vi "2100_SMU_Meas and Calculate Resitance_No Publish Data.vi"(7 "Current  Level":dbl=-0.01, 8 "error in (no error)":errorcluster, 10 "Pins":string[](array[string]), 11 "Semiconductor Module Context":T1) -> (0 "error Out":errorcluster, 1 "Individual_R_Meas":dbl[](array[numeric]), 3 "Semiconductor Module Context Out":T1)   [LabVIEW 2013]
uses:
  <vilib>/NI_TestStand_SemiconductorModule/NI_TestStand_Semiconductor_Module.lvlibp/PinMap/General/SemiconductorModuleContext.ctl
  <vilib>/NI_TestStand_SemiconductorModule/NI_TestStand_Semiconductor_Module.lvlibp/PinMap/DC Power/PinsToNIDCPowerSessions.vi
  <vilib>/NI_TestStand_SemiconductorModule/NI_TestStand_Semiconductor_Module.lvlibp
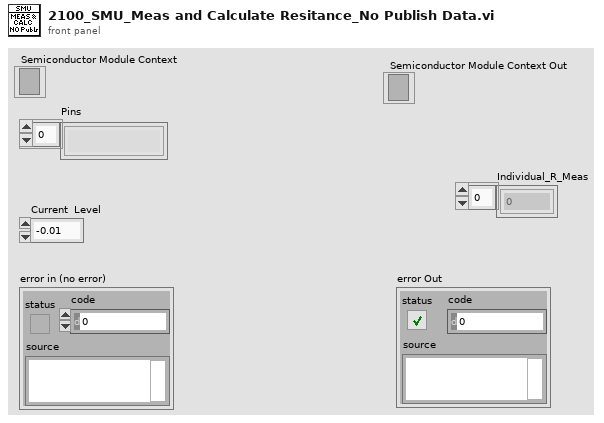
[diagram p1: front panel]
types:
  T1 = typedef "NI_TestStand_Semiconductor_Module.lvlibp/SemiconductorModuleContext.ctl" = refnum<k7>
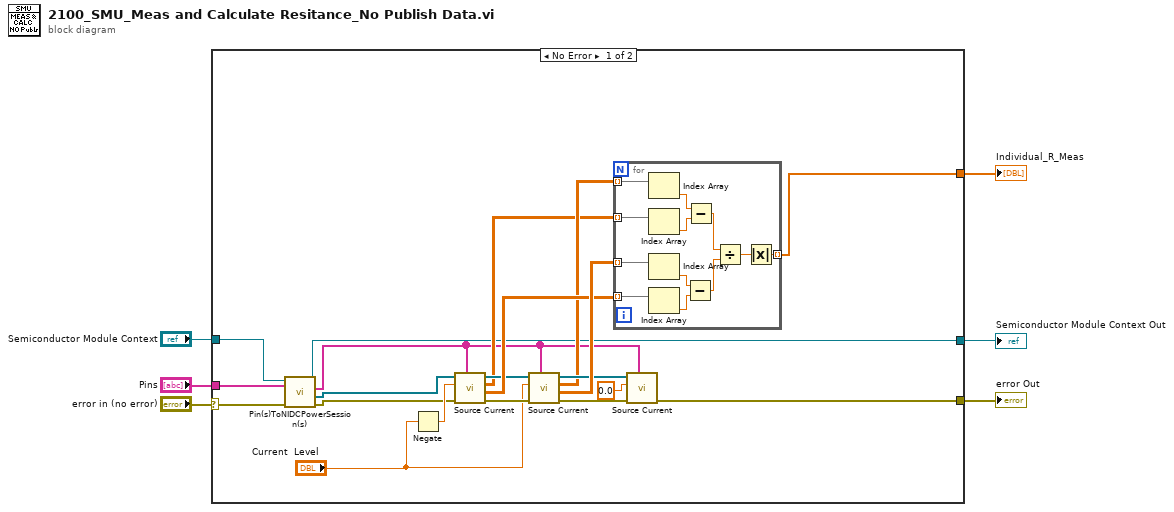
[diagram p0: block diagram]
diagram:
  n1 = case shown="No Error" "error in (no error)" {
    selector: "error in (no error)" -> [w26 w40]
    tunnel: "Semiconductor Module Context" -> [w24 w39]
    tunnel: "Pins" -> [w25 _]
    tunnel: [w10 w40] -> w3
    tunnel: [w9 w39] -> w2
    tunnel: [w7 _] -> w1
    frame No Error {
      n2 = call-poly <vilib>:"Pin(s)ToNIDCPowerSession(s).vi"("error in (no error)"=w26, "Pins"=w25, "Semiconductor Module Context"=w24) -> ("error out"=w12:errorcluster, "Instrument Sessions"=w11:refnum<k15>[], "Channel Lists"=w8:string[], "Semiconductor Module Context Out"=w9:T1)  [unwired: 4 in, 1 out]
      n3 = Negate(x="Current  Level") -> (-x=w20:dbl)
      n4 = call "Source Current.vi"("Channel Lists"=w8, "error in (no error)"=w12, "current level"=w20, "Instrument Sessions In"=w11) -> ("error out"=w18:errorcluster, "current measurements"=w22:dbl[][], "voltage measurements"=w16:dbl[][], "Instrument Sessions Out"=w17:refnum<k15>[])  [unwired: 4 in]
      n5 = call "Source Current.vi"("Channel Lists"=w8, "error in (no error)"=w18, "current level"="Current  Level", "Instrument Sessions In"=w17) -> ("error out"=w15:errorcluster, "current measurements"=w23:dbl[][], "voltage measurements"=w19:dbl[][], "Instrument Sessions Out"=w21:refnum<k15>[])  [unwired: 4 in]
      n6 = for {
        tunnel: w19 -> [w30] mode=indexing
        tunnel: w23 -> [w38] mode=indexing
        tunnel: [w36] -> w7 mode=indexing
        tunnel: w22 -> [w34] mode=indexing
        tunnel: w16 -> [w27] mode=indexing
        n7 = Index Array(array=w30) -> (element=w29:dbl)  [unwired: 1 in]
        n8 = Index Array(array=w27) -> (element=w28:dbl)  [unwired: 1 in]
        n9 = Index Array(array=w38) -> (element=w31:dbl)  [unwired: 1 in]
        n10 = Index Array(array=w34) -> (element=w33:dbl)  [unwired: 1 in]
        n11 = Subtract(x=w31, y=w33) -> (x-y=w32:dbl)
        n12 = Subtract(x=w29, y=w28) -> (x-y=w35:dbl)
        n13 = Divide(x=w35, y=w32) -> (x/y=w37:dbl)
        n14 = Absolute Value(x=w37) -> (abs(x)=w36:dbl)
      }
      n15 = call "Source Current.vi"("Channel Lists"=w8, "error in (no error)"=w15, "current level"=0.0, "Instrument Sessions In"=w21) -> ("error out"=w10:errorcluster)  [unwired: 4 in, 3 out]
    }
    frame Error {
    }
  }
  "error Out" <- w3
  "Semiconductor Module Context Out" <- w2
  "Individual_R_Meas" <- w1
